vi "VMI_set_Delay.vi"(7 "Try Card":bool, 8 "Error In":errorcluster, 10 "CmdStopDelay":refnum<vi>, 11 "Delay Cluster":T1={"System no."=0, "Identification"="", "Device ID out"=0, "Postion / mm"=[], "SN out"="", "Movement Range"=[], "Conn. Axes"=[], "Target Position / mm"=50.0, "Velocity / mm s^-1"=0.15, "Set-up"=FALSE, "Moving"=FALSE, "Step Size / mm "=0.15, "Stage Number"=0, "Polling Time /ms"=0, "Delay Scan?"=FALSE, "Accurate Scan"=FALSE, "CmdMovDelay"=FALSE, "CmdStopDelay"=FALSE, "Delay List"=[["Number", "Target / mm", "Relative Integration Time"]], "Scan Start /mm"=50.0, "Scan End / mm"=80.0, "Scan Velocity / mm s^-1"=0.15}) -> (0 "Error Out":errorcluster, 3 "Delay Cluster Out":T1={"System no."=0, "Identification"="", "Device ID out"=0, "Postion / mm"=[], "SN out"="", "Movement Range"=[], "Conn. Axes"=[], "Target Position / mm"=50.0, "Velocity / mm s^-1"=0.15, "Set-up"=FALSE, "Moving"=FALSE, "Step Size / mm "=0.15, "Stage Number"=0, "Polling Time /ms"=0, "Delay Scan?"=FALSE, "Accurate Scan"=FALSE, "CmdMovDelay"=FALSE, "CmdStopDelay"=FALSE, "Delay List"=[["Number", "Target / mm", "Relative Integration Time"]], "Scan Start /mm"=50.0, "Scan End / mm"=80.0, "Scan Velocity / mm s^-1"=0.15})   [LabVIEW 2018]
uses:
  Type defs/PI_delay_settings_alt.ctl
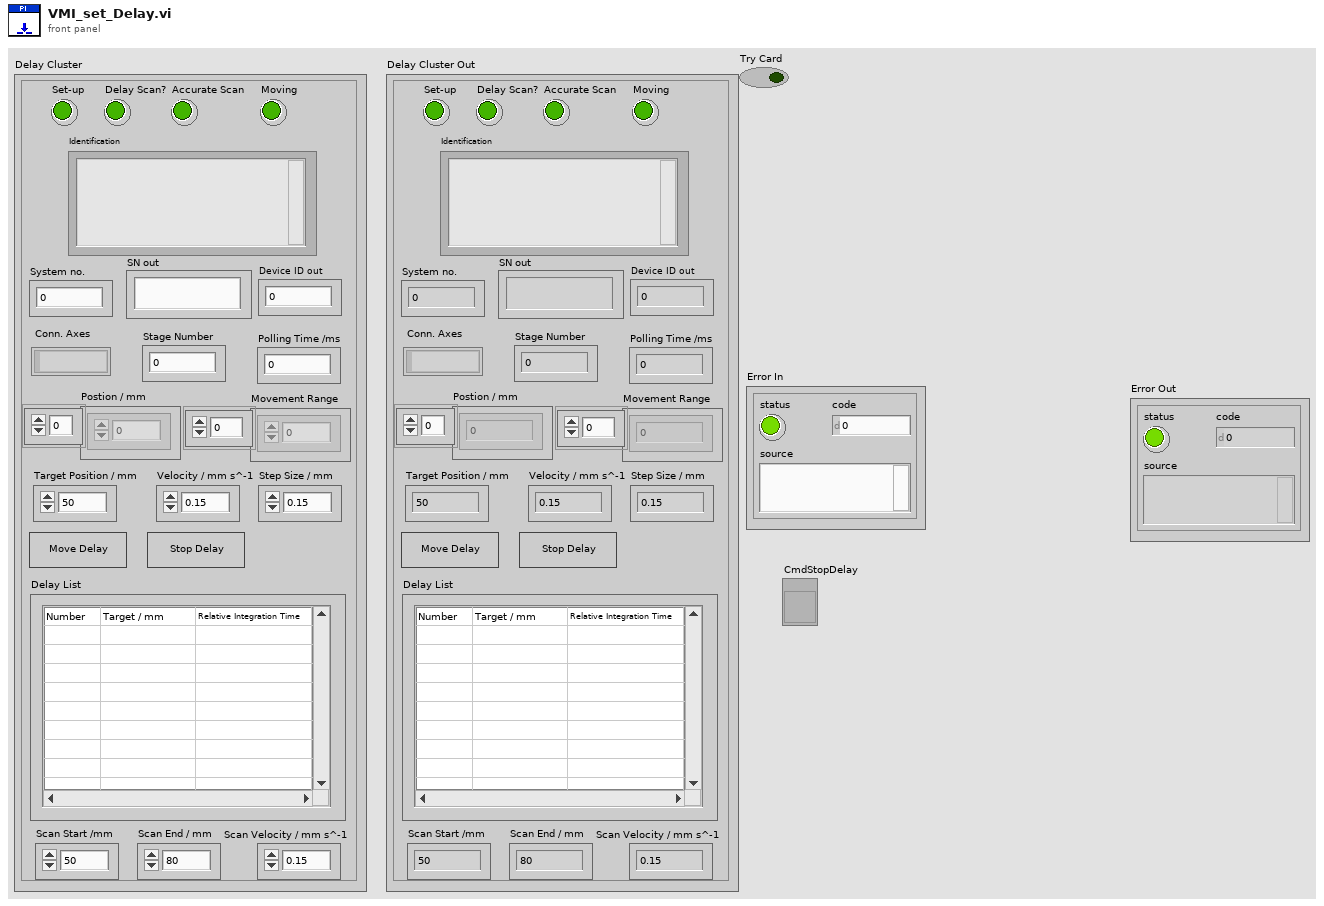
[diagram p1: front panel]
types:
  T1 = typedef "PI_delay_settings_alt.ctl" = cluster{"System no.":i32, "Identification":string, "Device ID out":i32, "Postion / mm":dbl[], "SN out":string, "Movement Range":dbl[], "Conn. Axes":string[], "Target Position / mm":dbl, "Velocity / mm s^-1":dbl, "Set-up":bool, "Moving":bool, "Step Size / mm ":dbl, "Stage Number":i32, "Polling Time /ms":i32, "Delay Scan?":bool, "Accurate Scan":bool, "CmdMovDelay":bool, "CmdStopDelay":bool, "Delay List":string[][], "Scan Start /mm":dbl, "Scan End / mm":dbl, "Scan Velocity / mm s^-1":dbl}
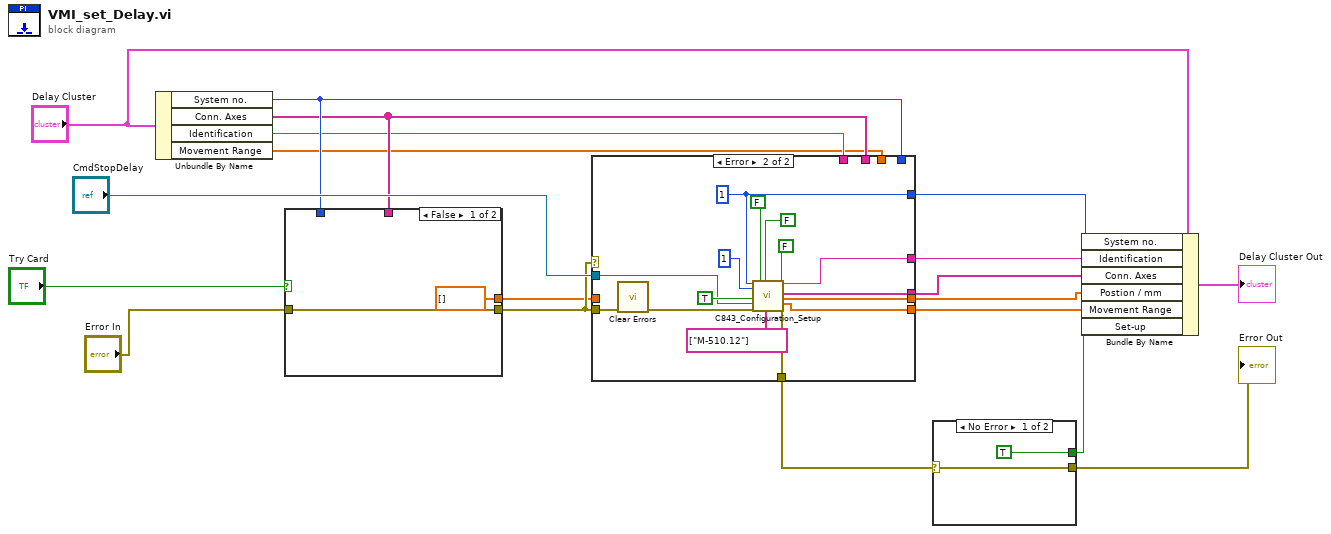
[diagram p0: block diagram]
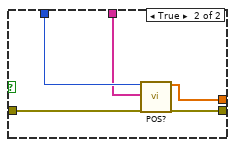
[diagram p2: hidden frame]
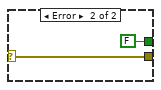
[diagram p4: hidden frame]
diagram:
  n1 = Unbundle By Name("Delay Cluster") -> ("System no."=w6:i32, "Conn. Axes"=w5:string[], "Identification"=w4:string, "Movement Range"=w2:dbl[])
  n2 = case shown="False" "Try Card" {
    tunnel: "Error In" -> [w21 w26]
    tunnel: [w21 w25] -> w7
    tunnel: w6 -> [_ w24]
    tunnel: w5 -> [_ w23]
    tunnel: [dbl[] [] ("Position") w22] -> w3
    frame False {
    }
    frame True {
      n3 = call "POS?.vi"("System no."=w24, "Axes to query"=w23, "error in"=w26) -> ("Position"=w22:dbl[], "error out"=w25:errorcluster)  [unwired: 2 in, 13 out]
    }
  }
  n4 = case shown="Error" w7 {
    tunnel: [w32 w42] -> w18
    tunnel: [w30 w41] -> w17
    tunnel: [w31 w40] -> w16
    tunnel: [w28 w39] -> w15
    tunnel: [w27 w38] -> w14
    tunnel: "CmdStopDelay" -> [_ w37]
    tunnel: [w29 w36] -> w10
    tunnel: w7 -> [w27 w35]
    tunnel: w6 -> [w32 _]
    tunnel: w5 -> [w31 _]
    tunnel: w4 -> [w30 _]
    tunnel: w3 -> [w29 _]
    tunnel: w2 -> [w28 _]
    frame No Error {
    }
    frame Error {
      w42 = 1 ("System no.")
      n5 = call <vilib>:"Clear Errors.vi"("error in (no error)"=w35) -> ("error out"=w34:errorcluster)  [unwired: 5 in, 1 out]
      n6 = call "C843_Configuration_Setup.vi"("System no."=w42, "C-843 Board No."=1, "All axes?"=TRUE, "Stop refnum"=w37, "error in"=w34, "C-843 version"=FALSE, "Use dialog to define\nconnected stages?"=FALSE ("Use dialog to define\nconnected stages?"), "Stage names input"=string[] ["M-510.12"], "Move to middle?"=FALSE) -> ("Identification"=w41:string, "Conn. \nAxes"=w40:string[], "Position"=w36:dbl[], "+/- movement\nrange"=w39:dbl[], "error out"=w38:errorcluster)  [unwired: 6 in]
    }
  }
  n7 = case shown="No Error" w14 {
    selector: w14 -> [w49 w51]
    tunnel: [w49 w51] -> w12
    tunnel: [TRUE FALSE] -> w13
    frame No Error {
    }
    frame Error {
    }
  }
  "Error Out" <- w12
  n8 = Bundle By Name(cluster="Delay Cluster", "System no."=w18, "Identification"=w17, "Conn. Axes"=w16, "Postion / mm"=w10, "Movement Range"=w15, "Set-up"=w13) -> (→"Delay Cluster Out":T1)
